vi "Editor.vi"(1 "File":path=path "C:/AzCam/systems/mont4k/FitsTemplates/FitsTemplate_mont4k_green.txt") -> (0 "error out":errorcluster)   [LabVIEW 2014]
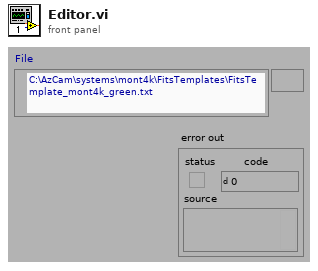
[diagram p1: front panel]
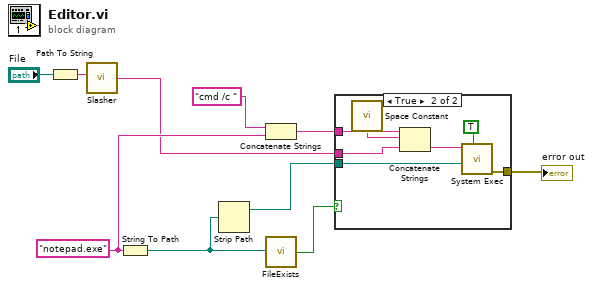
[diagram p0: block diagram]
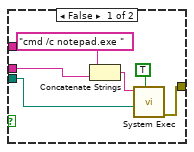
[diagram p2: hidden frame]
diagram:
  w5 = "notepad.exe" ("name or relative path")
  n1 = Path To String(path="File") -> (string=w4:string)
  n2 = call "Slasher.vi"("String In"=w4) -> ("String Out"=w3:string)
  n3 = String To Path(string=w5) -> (path=w6:path)
  n4 = Strip Path(path=w6) -> (stripped path=w9:path)  [unwired: 1 out]
  n5 = Concatenate Strings("cmd /c " ("name or relative path"), w5) -> (w8:string)
  n6 = call "FileExists.vi"("file path"=w6) -> ("Exists?"=w7:bool)
  n7 = case shown="True" w7 {
    tunnel: w8 -> [_ w21]
    tunnel: w9 -> [w13 w22]
    tunnel: w3 -> [w12 w18]
    tunnel: [w11 w17] -> w2
    frame False {
      n8 = Concatenate Strings("cmd /c notepad.exe " ("name or relative path"), w12) -> (w14:string)
      n9 = call <vilib>:"System Exec.vi"("wait until completion? (T)"=TRUE, "working directory"=w13, "command line"=w14) -> ("error out"=w11:errorcluster)  [unwired: 5 in, 3 out]
    }
    frame True {
      n10 = call <vilib>:"Space Constant.vi"() -> ("String"=w19:string)
      n11 = Concatenate Strings(w21, w19, w18) -> (w20:string)
      n12 = call <vilib>:"System Exec.vi"("wait until completion? (T)"=TRUE, "working directory"=w22, "command line"=w20) -> ("error out"=w17:errorcluster)  [unwired: 5 in, 3 out]
    }
  }
  "error out" <- w2
